vi "Calibrate.vi"(11 "Connection Cluster in":T1) -> (3 "Connection Cluster out":T1)   [LabVIEW 2013]
panel:
  out "element":dbl
  out "Array":dbl[][](array[numeric])
  out "Waveform Graph":waveform(dbl)(graph)
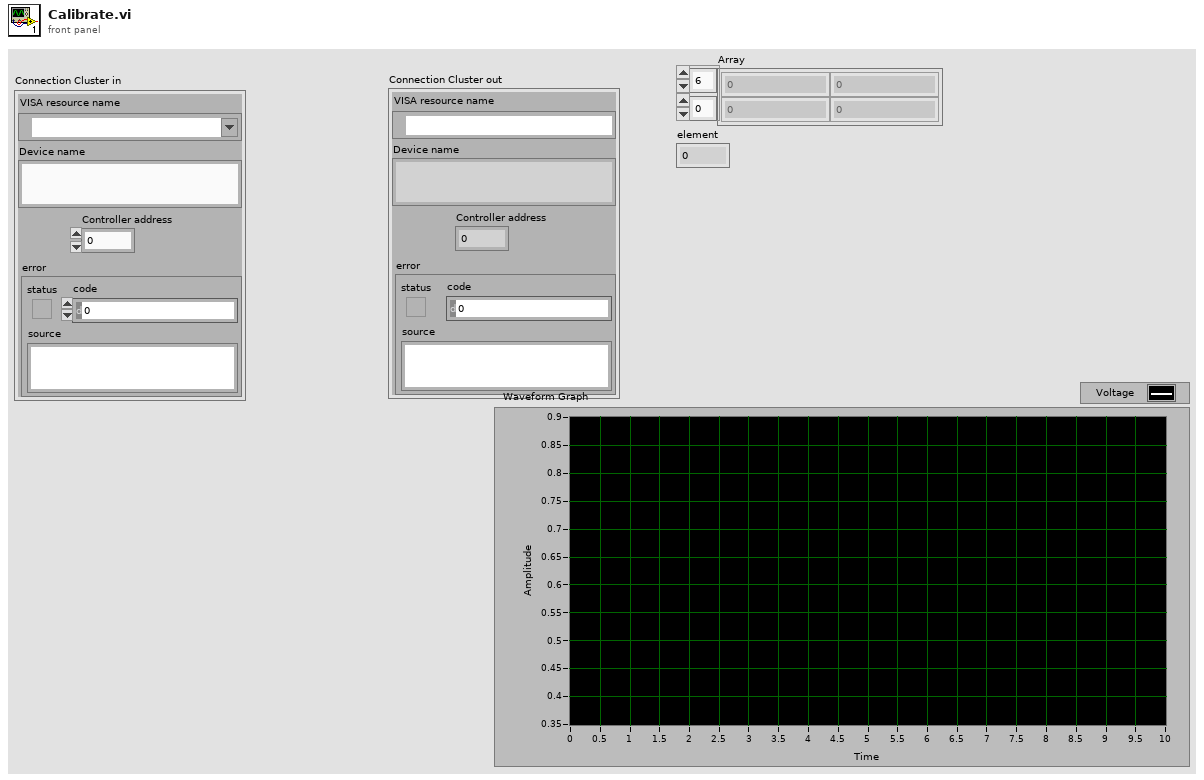
[diagram p1: front panel]
types:
  T1 = cluster{"VISA resource name":refnum<visa-resource-name>, "Device name":string, "Controller address":i32, "error":errorcluster}
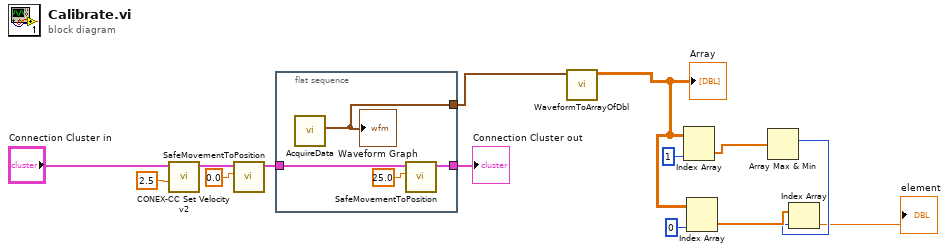
[diagram p0: block diagram]
diagram:
  n1 = call <userlib>:"CONEX-CC Set Velocity v2.vi"("Velocity"=2.5, "Connection Cluster in"="Connection Cluster in") -> ("Connection Cluster out"=w12:T1)  [unwired: 9 in]
  n2 = call "SafeMovementToPosition.vi"("Target position"=0.0, "Connection Cluster in"=w12) -> ("Connection Cluster out"=w10:T1)  [unwired: 9 in]
  n3 = flat-sequence {
    tunnel: w10 -> [w18]
    tunnel: [w16] -> w9
    tunnel: [w15] -> w8
    frame #0 {
      n4 = call "AcquireData.vi"() -> ("data"=w15:waveform(dbl))  [unwired: 9 in, 2 out]
      "Waveform Graph" <- w15
      n5 = call "SafeMovementToPosition.vi"("Target position"=25.0, "Connection Cluster in"=w18) -> ("Connection Cluster out"=w16:T1)  [unwired: 9 in]
    }
  }
  n6 = call "WaveformToArrayOfDbl.vi"("waveform"=w8) -> ("Array"=w5:dbl[][])  [unwired: 10 in]
  "Array" <- w5
  n7 = Index Array(array=w5, index (col)=1 ("disabled index (col)")) -> (element=w6:dbl[])  [unwired: 1 in]
  n8 = Index Array(array=w5, index (col)=0 ("disabled index (col)")) -> (element=w3:dbl[])  [unwired: 1 in]
  n9 = Array Max & Min(array=w6) -> (max index (indices)=w2:i32)  [unwired: 3 out]
  n10 = Index Array(array=w3, index=w2) -> (element=→"element":dbl)
  "Connection Cluster out" <- w9
